vi "aaa2.vi"() -> ()   [LabVIEW 2010]
panel:
  out "filenames":string[](array[string])
  out "time string":string
  out "date string":string
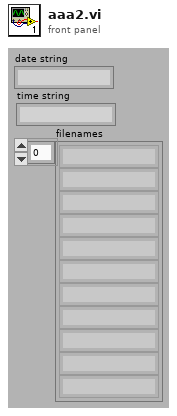
[diagram p1: front panel]
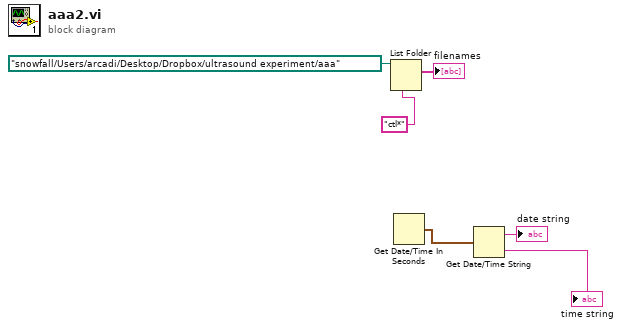
[diagram p0: block diagram]
diagram:
  n1 = List Folder(path=path "/snowfall/Users/arcadi/Desktop/Dropbox/ultrasound experiment/aaa", pattern="ctl*") -> (filenames=→"filenames":string[])  [unwired: 2 in, 3 out]
  n2 = Get Date/Time In Seconds() -> (seconds since 1Jan1904=w6:timestamp)
  n3 = Get Date/Time String(seconds (now)=w6) -> (date string=→"date string":string, time string=→"time string":string)  [unwired: 2 in]
